vi "Update parameters (polymorphic).vi"   [LabVIEW 2020, in "Measurement.lvclass"]
uses:
  Measurement.lvclass
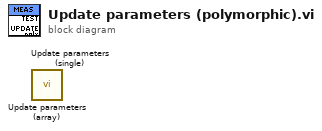
[diagram p0: block diagram]
diagram:
  n1 = call "Update parameters (array).vi"() -> ()  [unwired: 11 in, 1 out]
  n2 = call "Update parameters (single).vi"() -> ()  [unwired: 11 in, 1 out]
